vi "CheckCanComm.vi"(1 "类型":u32(ring)=4 items=["PCI5121"=1, "PCI9810"=2, "USBCAN1"=3, "USBCAN2"=4, "PCI9820"=5, "CAN232"=6, "PCI5110"=7, "CANLite(mini)"=8, "ISA9620"=9, "ISA5420"=10, "PC104CAN"=11, "CANET"=17, "DNP9810"=13, "USBCAN-E-U"=20, "USBCAN-2E-U"=21], 2 "设备索引":u32(ring) items=["0", "1", "2", "3", "4", "5", "6", "7", "8", "9", "10", "11", "12", "13", "14", "15", ""], 3 "CAN路数":u32(ring) items=["0", "1"], 11 "time out":u32) -> (4 "recv ok?":bool)   [LabVIEW 2013]
uses:
  BMS_BootLoader/trunk/BMS_Bootloader/AutoBurn/Settings/ControlCAN.dll
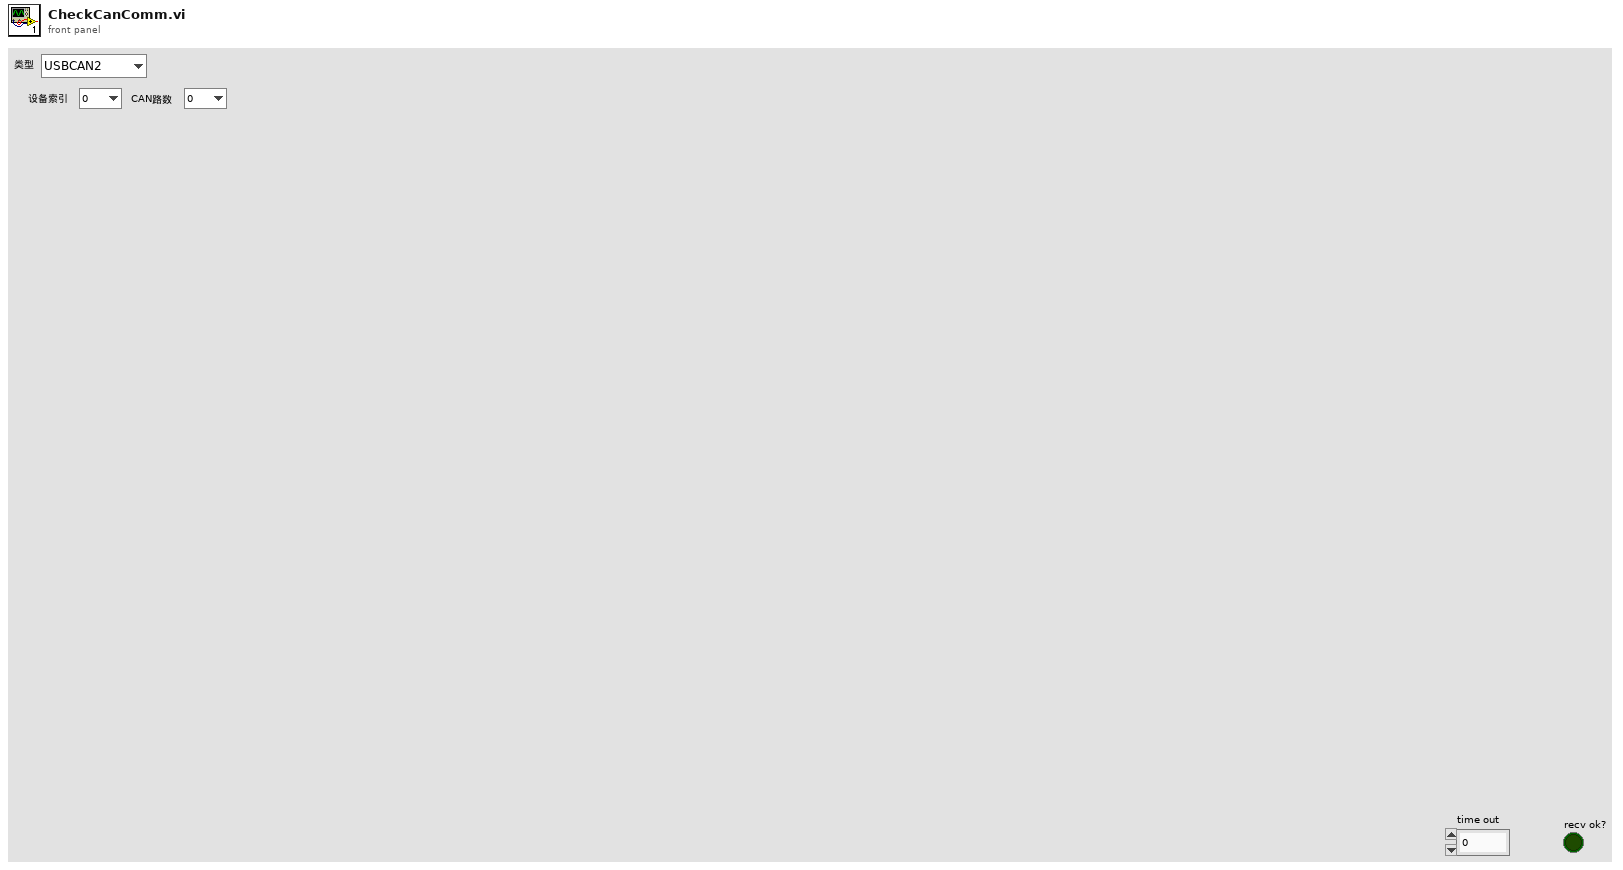
[diagram p1: front panel]
types:
  T1 = cluster{"ID":u32, "TimeStamp":u32, "TimeFlag":u8, "SendType":u8, "RemoteFlag":u8, "ExternFlag":u8, "DataLen":u8, u8, u8, u8, u8, u8, u8, u8, u8, u8, u8, u8}
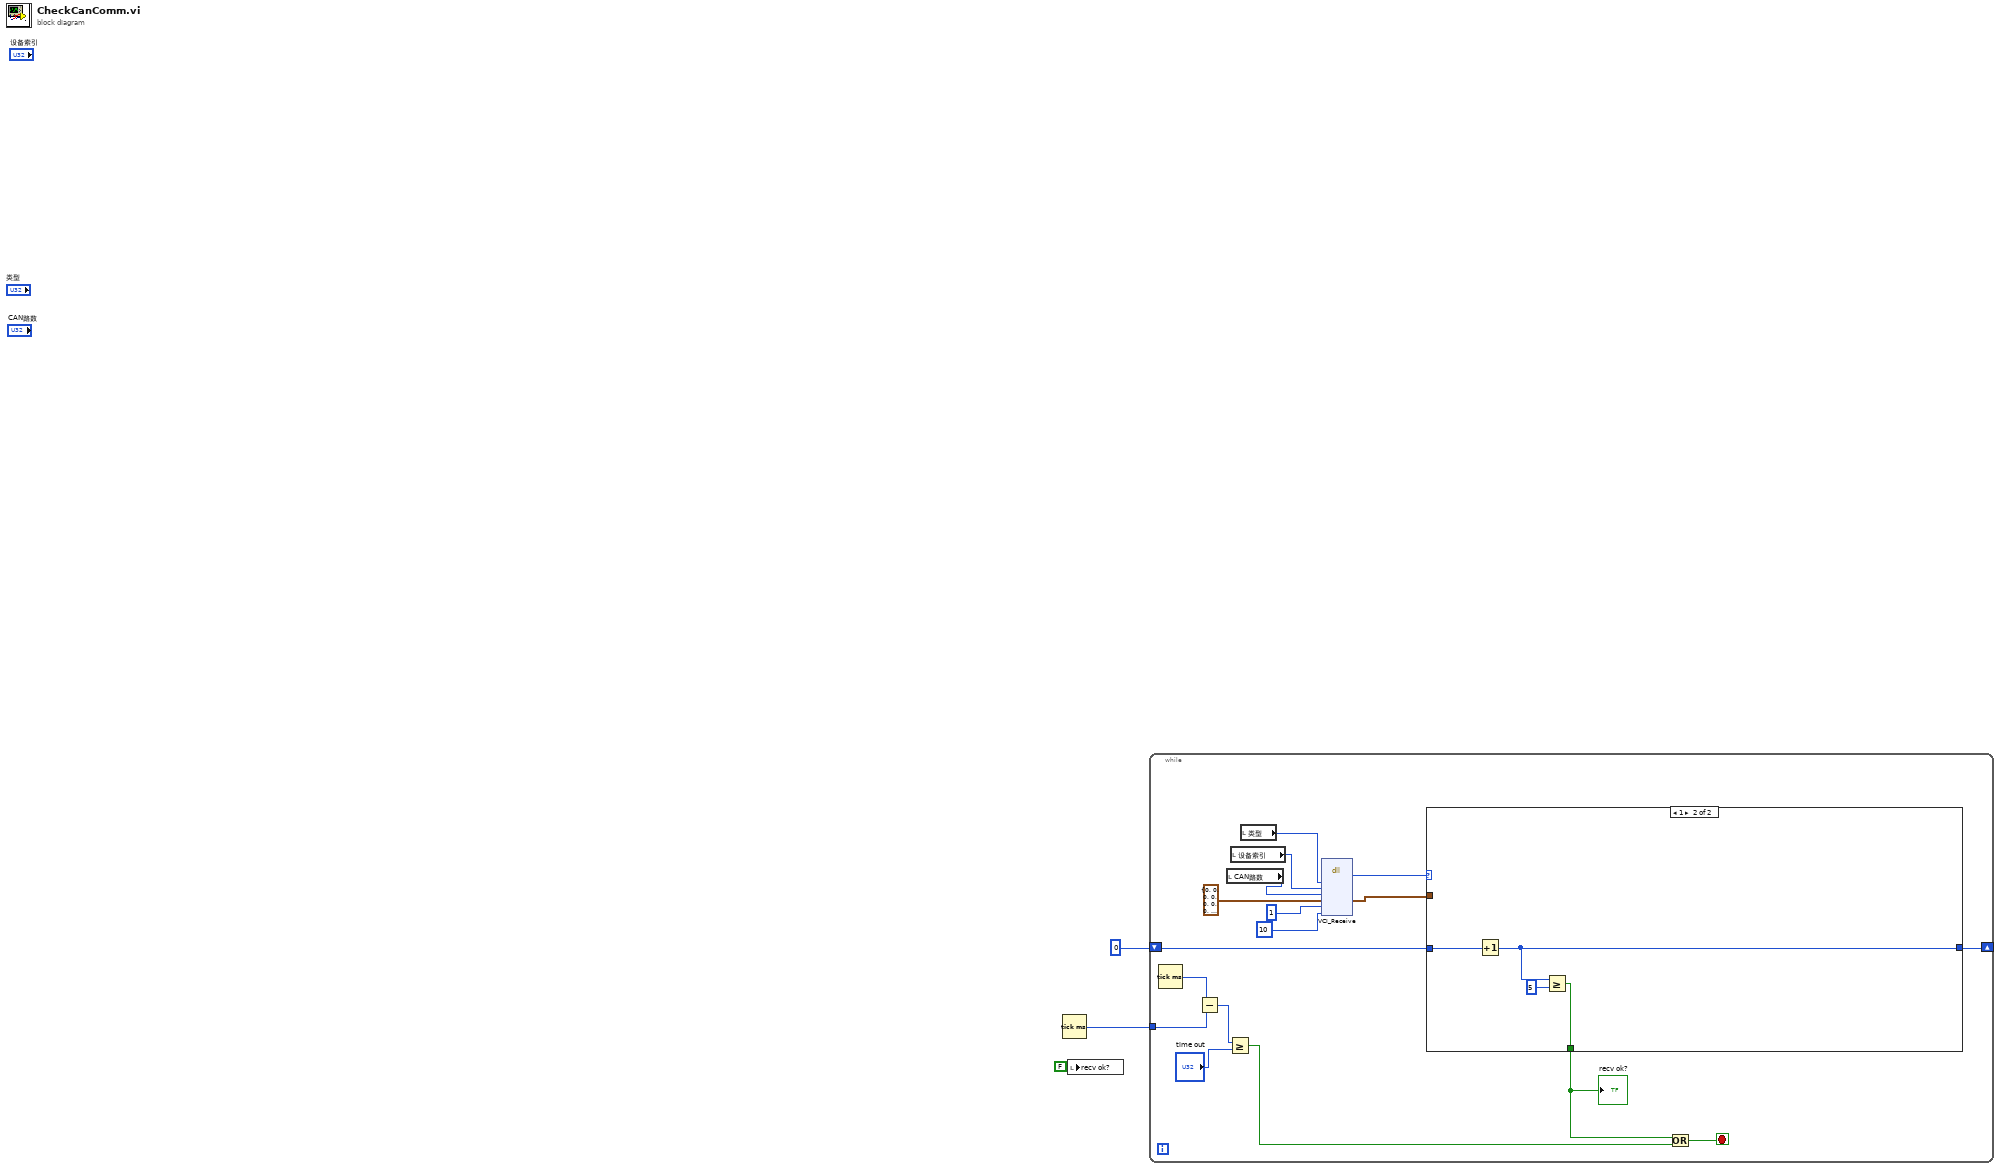
[diagram p0: block diagram]
diagram:
  n1 = Tick Count (ms)() -> (millisecond timer value=w3:u32)
  n2 = local write "recv ok?"(FALSE ("x = y?")) -> ()
  n3 = while {
    tunnel: w3 -> [w13]
    shift-right: [w5] -> _
    shift-left: u8 0 ("times") -> [w6]
    stop <- w9 stop-if-true
    n4 = Tick Count (ms)() -> (millisecond timer value=w14:u32)
    n5 = Subtract(x=w14, y=w13) -> (x-y=w12:u32)
    n6 = local read "CAN路数"() -> (w18:u32)
    n7 = Greater Or Equal?(x=w12, y="time out") -> (x >= y?=w10:bool)
    n8 = local read "设备索引"() -> (w15:u32)
    n9 = local read "类型"() -> (w16:u32)
    n10 = dll-call lib="F:/Bluewave New Energy/SVN_Work/BMS_BootLoader/trunk/BMS_Bootloader/AutoBurn/Settings/ControlCAN.dll" fn="VCI_Receive"("DeviceType"=w16, "DeviceInd"=w15, "CANInd"=w18, "pReceive"=T1 {"ID"=0, "TimeStamp"=0, "TimeFlag"=0, "SendType"=0, "RemoteFlag"=0, "ExternFlag"=0, "DataLen"=0, 0, 0, 0, 0, 0, 0, 0, 0, 0, 0, 0}, "Len"=u32 1, "WaitTime"=10) -> ("返回类型"=w7:u32, "pReceive"=w8:T1)  [unwired: 8 in, 2 out]
    n11 = case shown="1" w7 {
      tunnel: w8 -> [_ _]
      tunnel: w6 -> [w21 w25]
      tunnel: [w21 w24] -> w5
      tunnel: [_ w22] -> w4
      frame 0, Default {
      }
      frame 1 {
        n12 = Increment(x=w25) -> (x+1=w24:u8)
        n13 = Greater Or Equal?(x=w24, y=u8 5) -> (x >= y?=w22:bool)
      }
    }
    "recv ok?" <- w4
    n14 = Or(x=w4, y=w10) -> (x .or. y?=w9:bool)
  }
